vi "Array Get Element At (Dimensions).vi"(8 "error in (no error)":errorcluster, 10 "Index":i32[](array[numeric]), 11 "Array DVR in":refnum<data-value>) -> (0 "error out":errorcluster, 2 "Element out":refnum<data-value>, 3 "Array DVR out":refnum<data-value>)   [LabVIEW 2012, in "MDSplus.lvlib"]
doc: "Return a single element, if the passed number of dimension is equals to the dimension of dims field. Otherwise it returns the reshaped array corresponding to the passed dimension array. For example, if the array is bi-dimensional, a single dimension i will specify the i-th row.\nNote that this method may be implemented at this level since ArrayData has all the required information about data and dimension."
uses:
  <vilib>/MDSplus/Library/MDSplus.lvlib
  <vilib>/MDSplus/Classes/Data_Class/Array_Class/Array.lvclass
  <vilib>/MDSplus/Classes/Data_Class/Data.lvclass
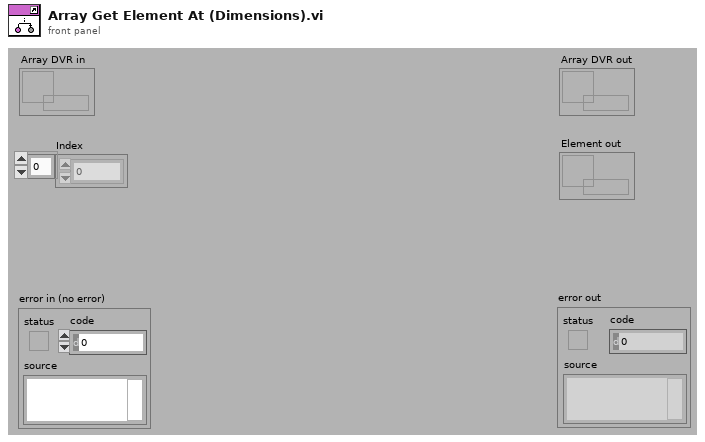
[diagram p1: front panel]
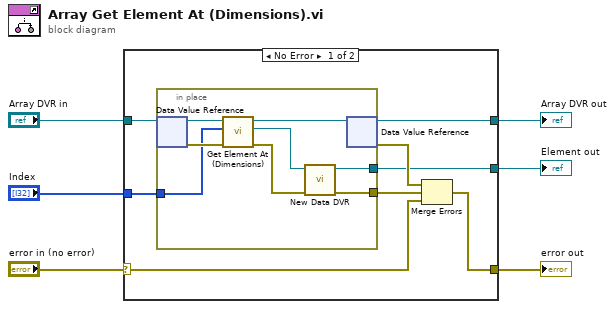
[diagram p0: block diagram]
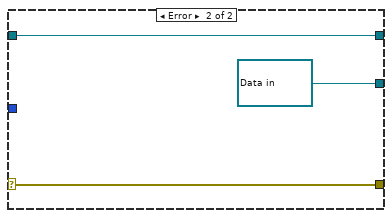
[diagram p2: hidden frame]
diagram:
  n1 = case shown="No Error" "error in (no error)" {
    selector: "error in (no error)" -> [w12 w25]
    tunnel: "Array DVR in" -> [w14 w24]
    tunnel: [w10 w25] -> w6
    tunnel: [w9 w24] -> w3
    tunnel: "Index" -> [w8 _]
    tunnel: [w7 refnum<data-value> refnum ("Data DVR out")] -> w1
    frame No Error {
      n2 = in-place {
        in-place-border: [w16] -> w13
        in-place-border: w8 -> [w19]
        in-place-border: [w15] -> w7
        n3 = in-place-dvr #1(w14) -> (w22:refnum<class "Array.lvclass">, w20:errorcluster)
        n4 = call-dynamic "Get Element At (Dimensions).vi"("error in (no error)"=w20, "Index"=w19, "Array in"=w22) -> ("error out"=w17:errorcluster, "Element out"=w18:refnum<class "Data.lvclass">, "Array out"=w21:refnum<class "Array.lvclass">)  [unwired: 6 in]
        n5 = call <vilib>:"New Data DVR.vi"("error in (no error)"=w17, "Data in"=w18) -> ("error out"=w16:errorcluster, "Data DVR out"=w15:refnum<data-value>)  [unwired: 8 in]
        n6 = in-place-dvr #1(w21) -> (w9:refnum<data-value>, w11:errorcluster)
      }
      n7 = Merge Errors(w11, w13, w12) -> (w10:errorcluster)
    }
    frame Error {
    }
  }
  "error out" <- w6
  "Array DVR out" <- w3
  "Element out" <- w1
